vi "DLLpathGloabl.vi"(10 "DLLpath":path, 11 "Set/Get":bool) -> (3 "PathOut":path)   [LabVIEW 2014]
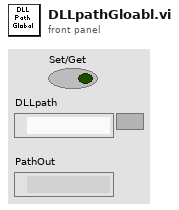
[diagram p1: front panel]
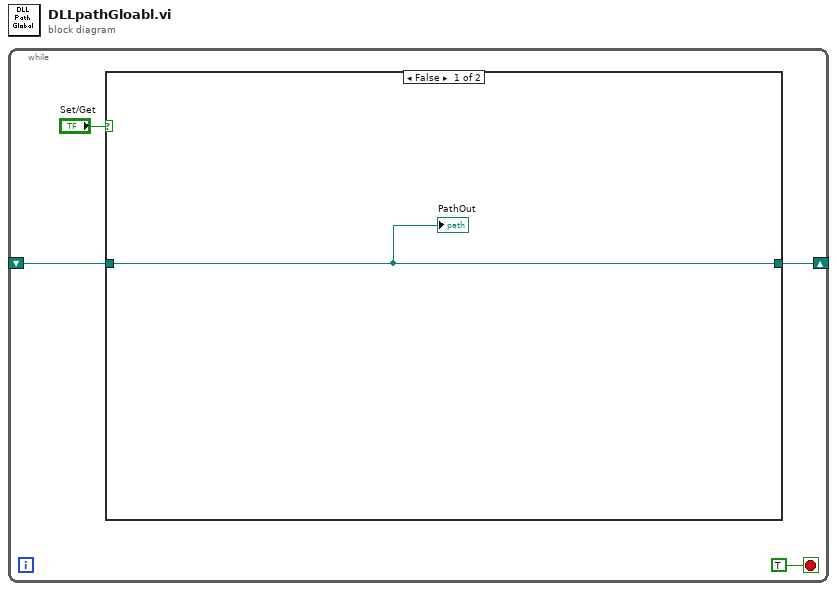
[diagram p0: block diagram]
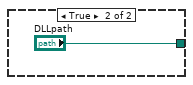
[diagram p2: hidden frame]
diagram:
  n1 = while {
    shift-right: [w2] -> _
    shift-left: _ -> [w1]
    stop <- TRUE stop-if-true
    n2 = case shown="False" "Set/Get" {
      tunnel: [w5 "DLLpath"] -> w2
      tunnel: w1 -> [w5 _]
      frame False {
        "PathOut" <- w5
      }
      frame True {
      }
    }
  }
